vi "Recurse Structure Objects.vi"(11 "Objects In":refnum<vi>[](array[refnum])) -> (3 "Objects Out":refnum<vi>[](array[refnum]))   [LabVIEW 2019]
doc: "Return all the objects within a given structure, including those in sub-structures. Only objects in the currently visible frame are included. Decoration objects and the structures themselves are excluded from the resulting object list."
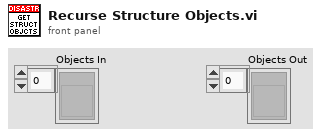
[diagram p1: front panel]
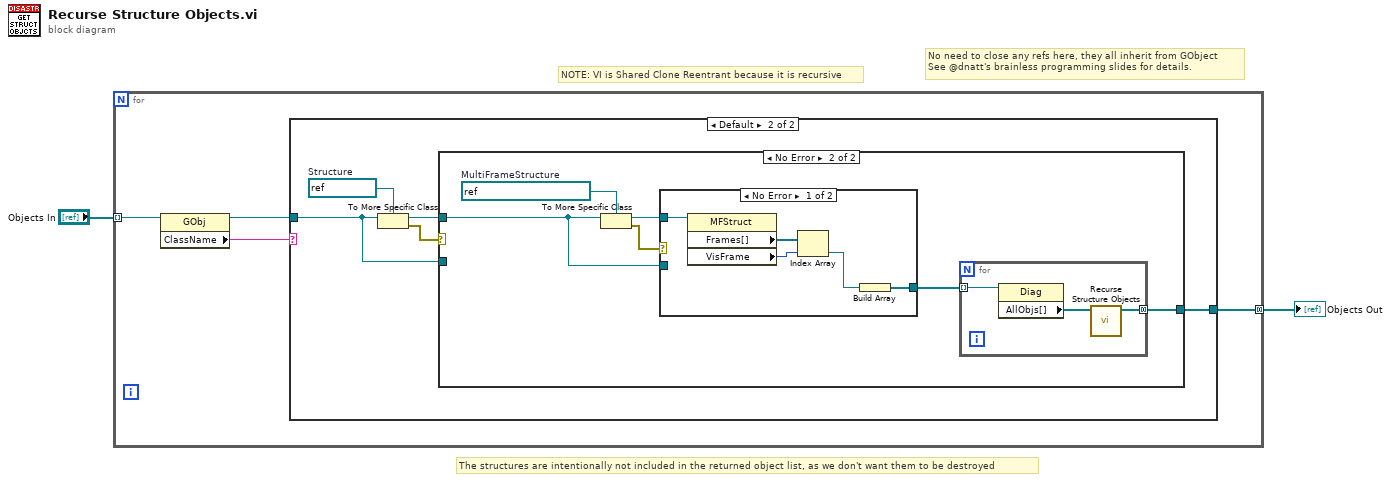
[diagram p0: block diagram]
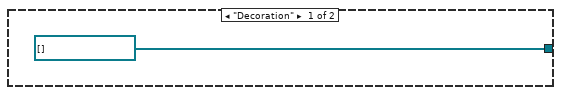
[diagram p2: hidden frame]
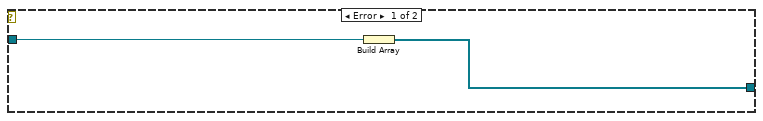
[diagram p3: hidden frame]
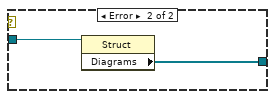
[diagram p4: hidden frame]
diagram:
  # "No need to close any refs here, they all inherit from GObject\nSee @dnatt's brainless programming slides for details."
  # "NOTE: VI is Shared Clone Reentrant because it is recursive"
  # "The structures are intentionally not included in the returned object list, as we don't want them to be destroyed"
  n1 = for {
    tunnel: "Objects In" -> [w4] mode=indexing
    tunnel: [w6] -> w1 mode=concatenating
    n2 = property class="GObj"(reference=w4) -> (reference out=w5:refnum<vi>, "ClassName"=w3:string)  [unwired: 1 in, 1 out]
    n3 = case shown="Default" w3 {
      tunnel: [refnum<vi>[] [] ("Object Out") w9] -> w6
      tunnel: w5 -> [_ w8]
      frame "Decoration" {
      }
      frame Default {
        w12 = refnum<vi> refnum  # Structure
        n4 = To More Specific Class(target class=w12, reference=w8) -> (specific class reference=w11:refnum<vi>, error out=w10:errorcluster)  [unwired: 1 in]
        n5 = case shown="No Error" w10 {
          tunnel: w11 -> [_ w16]
          tunnel: w8 -> [w14 _]
          tunnel: [w13 w20] -> w9
          frame Error {
            n6 = Build Array(w14) -> (w13:refnum<vi>[])
          }
          frame No Error {
            w19 = refnum<vi> refnum  # MultiFrameStructure
            n7 = To More Specific Class(target class=w19, reference=w16) -> (specific class reference=w17:refnum<vi>, error out=w18:errorcluster)  [unwired: 1 in]
            n8 = case shown="No Error" w18 {
              tunnel: w17 -> [w25 _]
              tunnel: w16 -> [_ w27]
              tunnel: [w21 w26] -> w15
              frame No Error {
                n9 = property class="MFStruct"(reference=w25) -> ("Frames[]"=w24:refnum<vi>[], "VisFrame"=w23:u32)  [unwired: 1 in, 2 out]
                n10 = Index Array(array=w24, index=w23) -> (element=w22:refnum<vi>)
                n11 = Build Array(w22) -> (w21:refnum<vi>[])
              }
              frame Error {
                n12 = property class="Struct"(reference=w27) -> ("Diagrams"=w26:refnum<vi>[])  [unwired: 1 in, 2 out]
              }
            }
            n13 = for {
              tunnel: w15 -> [w30] mode=indexing
              tunnel: [w28] -> w20 mode=concatenating
              n14 = property class="Diag"(reference=w30) -> ("AllObjs[]"=w29:refnum<vi>[])  [unwired: 1 in, 2 out]
              n15 = call "Recurse Structure Objects.vi"("Objects In"=w29) -> ("Objects Out"=w28:refnum<vi>[])  [unwired: 10 in]
            }
          }
        }
      }
    }
  }
  "Objects Out" <- w1
